vi "난수45.vi"() -> ()   [LabVIEW 2014]
panel:
  out "웨이브폼 차트":dbl(graph)
  out "ceil(x): 가장 작은 정수 >= x":dbl
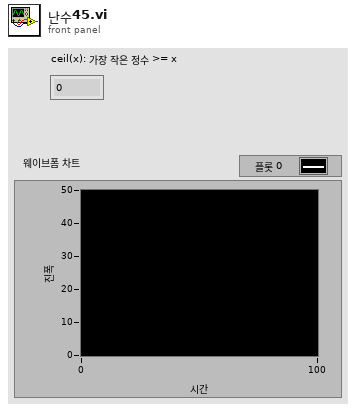
[diagram p1: front panel]
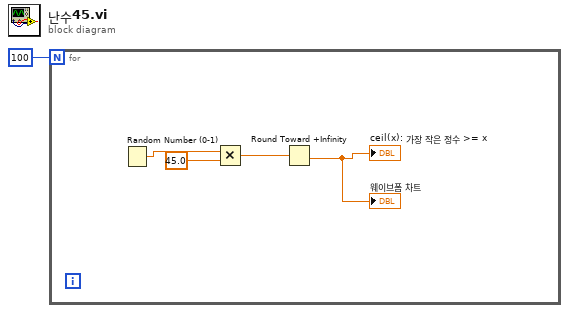
[diagram p0: block diagram]
diagram:
  n1 = for {
    N: 100 -> [_]
    n2 = Random Number (0-1)() -> (number: 0 to 1=w5:dbl)
    n3 = Multiply(x=w5, y=45.0) -> (x*y=w3:dbl)
    n4 = Round Toward +Infinity(x=w3) -> (ceil(x): smallest int >= x=→"ceil(x): 가장 작은 정수 >= x" →"웨이브폼 차트":dbl)
  }
